vi "CRYDelete Tree Items.vi"(10 "Array":i32[](array[numeric]), 11 "Type":enum16{"Curves", "Values", "Results", "WFM"}(ring)) -> ()   [LabVIEW 2013]
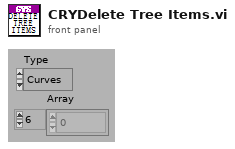
[diagram p1: front panel]
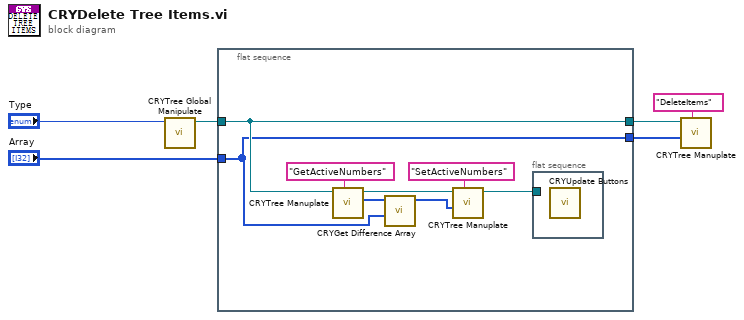
[diagram p0: block diagram]
diagram:
  n1 = call "CRYTree Global Manipulate.vi"("Type In"="Type") -> ("Tree/Curve Tree"=w4:refnum<vi>)  [unwired: 7 in, 3 out]
  n2 = flat-sequence {
    tunnel: w4 -> [w9]
    tunnel: "Array" -> [w8]
    tunnel: [w9] -> w3
    tunnel: [w8] -> w2
    frame #0 {
      n3 = call "CRYTree Manuplate.vi"("sAction"="GetActiveNumbers", "Tree in"=w9) -> ("nData Out"=w13:i32[], "Tree Out"=w11:refnum<vi>)  [unwired: 6 in, 2 out]
      n4 = call "CRYGet Difference Array.vi"("Array 2"=w8, "Array 1"=w13) -> ("Diff Out"=w10:i32[])  [unwired: 8 in, 1 out]
      n5 = call "CRYTree Manuplate.vi"("sAction"="SetActiveNumbers", "nData"=w10, "Tree in"=w11) -> ("Tree Out"=w7:refnum<vi>)  [unwired: 5 in, 3 out]
      n6 = flat-sequence {
        tunnel: w7 -> [_]
        frame #0 {
          n7 = call "CRYUpdate Buttons.vi"() -> ()  [unwired: 12 in]
        }
      }
    }
  }
  n8 = call "CRYTree Manuplate.vi"("sAction"="DeleteItems", "nData"=w2, "Tree in"=w3) -> ()  [unwired: 5 in, 4 out]
